vi "Fdx Write (UDP-SAP).vi"(6 "IpDst":u32, 7 "UdpDst":u32, 8 "error in (no error)":errorcluster, 9 "Data":u8[](array[numeric]) format="%.0x", 10 "UdpHandle in":u32, 11 "InstrumentHandle_port in":u32) -> (0 "error out":errorcluster, 1 "BytesWritten":u32, 2 "UdpHandle out":u32, 3 "InstrumentHandle_port out":u32)   [LabVIEW 2020, in "AIM664LV.lvlib"]
uses:
  AIM664LV.lvlib
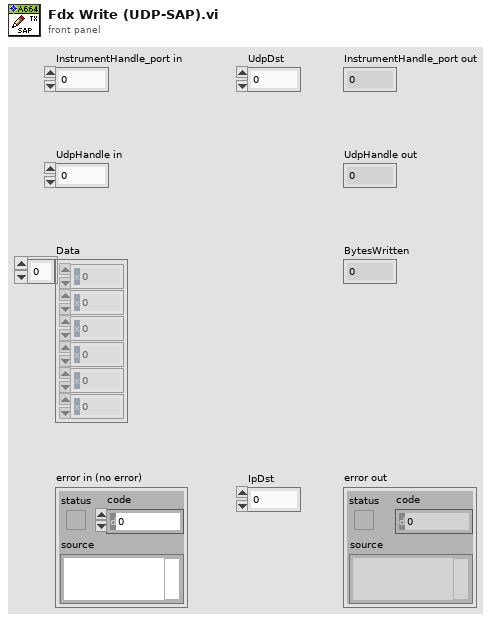
[diagram p1: front panel]
types:
  T1 = cluster{"UdpHandle":u32, "UdpDst":u32, "IpDst":u32, "ByteCount":u32, "Data":u8[]}
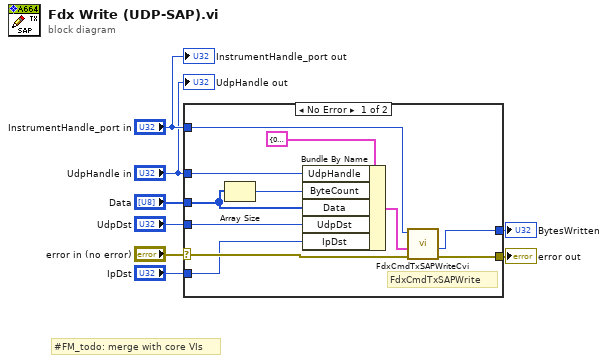
[diagram p0: block diagram]
diagram:
  # "#FM_todo: merge with core VIs"
  n1 = case shown="No Error" "error in (no error)" {
    selector: "error in (no error)" -> [w19 w20]
    tunnel: [w18 w20] -> w7
    tunnel: "Data" -> [w14 _]
    tunnel: "IpDst" -> [w13 _]
    tunnel: "UdpDst" -> [w12 _]
    tunnel: [w11 _] -> w3
    tunnel: "InstrumentHandle_port in" -> [w10 _]
    tunnel: "UdpHandle in" -> [w9 _]
    frame No Error {
      # "FdxCmdTxSAPWrite"
      n2 = Array Size(array=w14) -> (size(s)=w15:i32)
      n3 = Bundle By Name(cluster=T1 {"UdpHandle"=0, "UdpDst"=0, "IpDst"=0, "ByteCount"=0, "Data"=[]} ("TxSapWriteIn"), "UdpHandle"=w9, "ByteCount"=w15, "Data"=w14, "UdpDst"=w12, "IpDst"=w13) -> (w16:T1)
      n4 = call "FdxCmdTxSAPWriteCvi.vi"("error in"=w19, "TxSapWriteIn"=w16, "InstrumentHandle"=w10) -> ("error out"=w18:errorcluster, "BytesWritten"=w11:u32)  [unwired: 6 in, 1 out]
    }
    frame Error {
    }
  }
  "error out" <- w7
  "BytesWritten" <- w3
  "InstrumentHandle_port out" <- "InstrumentHandle_port in"
  "UdpHandle out" <- "UdpHandle in"
